vi "Final Project.vi"() -> ()   [LabVIEW 2022 SP3]
uses:
  <vilib>/Analysis/3filter.llb/Filter Passband Type.ctl
  <vilib>/Instr/_visa.llb/VISA Configure Serial Port (Instr).vi
  <vilib>/ptbypt/NI_PtbyPt.lvlib
  <vilib>/Analysis/NI_AALBase.lvlib
panel:
  out "EMG2":dbl
  out "EMG1":dbl
  in  "stop 3":bool
  out "Raw Data File":refnum<file>
  in  "stop 2":bool
  out "Folder_Name":string
  out "Jump Indicator":bool
  out "Jump Binary":dbl(graph)
  out "Left Indicator":bool
  out "Move Left Binary":dbl(graph)
  out "Voltage (Analog) 2":dbl(graph)
  out "Right Indicator":bool
  out "Move Right Binary":dbl(graph)
  out "Voltage (Analog)":dbl(graph)
  out "number":u32
  out "Index":i32
  out "read buffer":string
  out "Serial Settings:Number of Bytes at Serial Port":u32
  in  "stop":bool
  out "Available?":bool
  out "string":string
  in  "Knob":dbl(knob) scale=0.0..2.0
  in  "VISA resource name":refnum<visa-resource-name>
  in  "Baud Rate":u32=9600
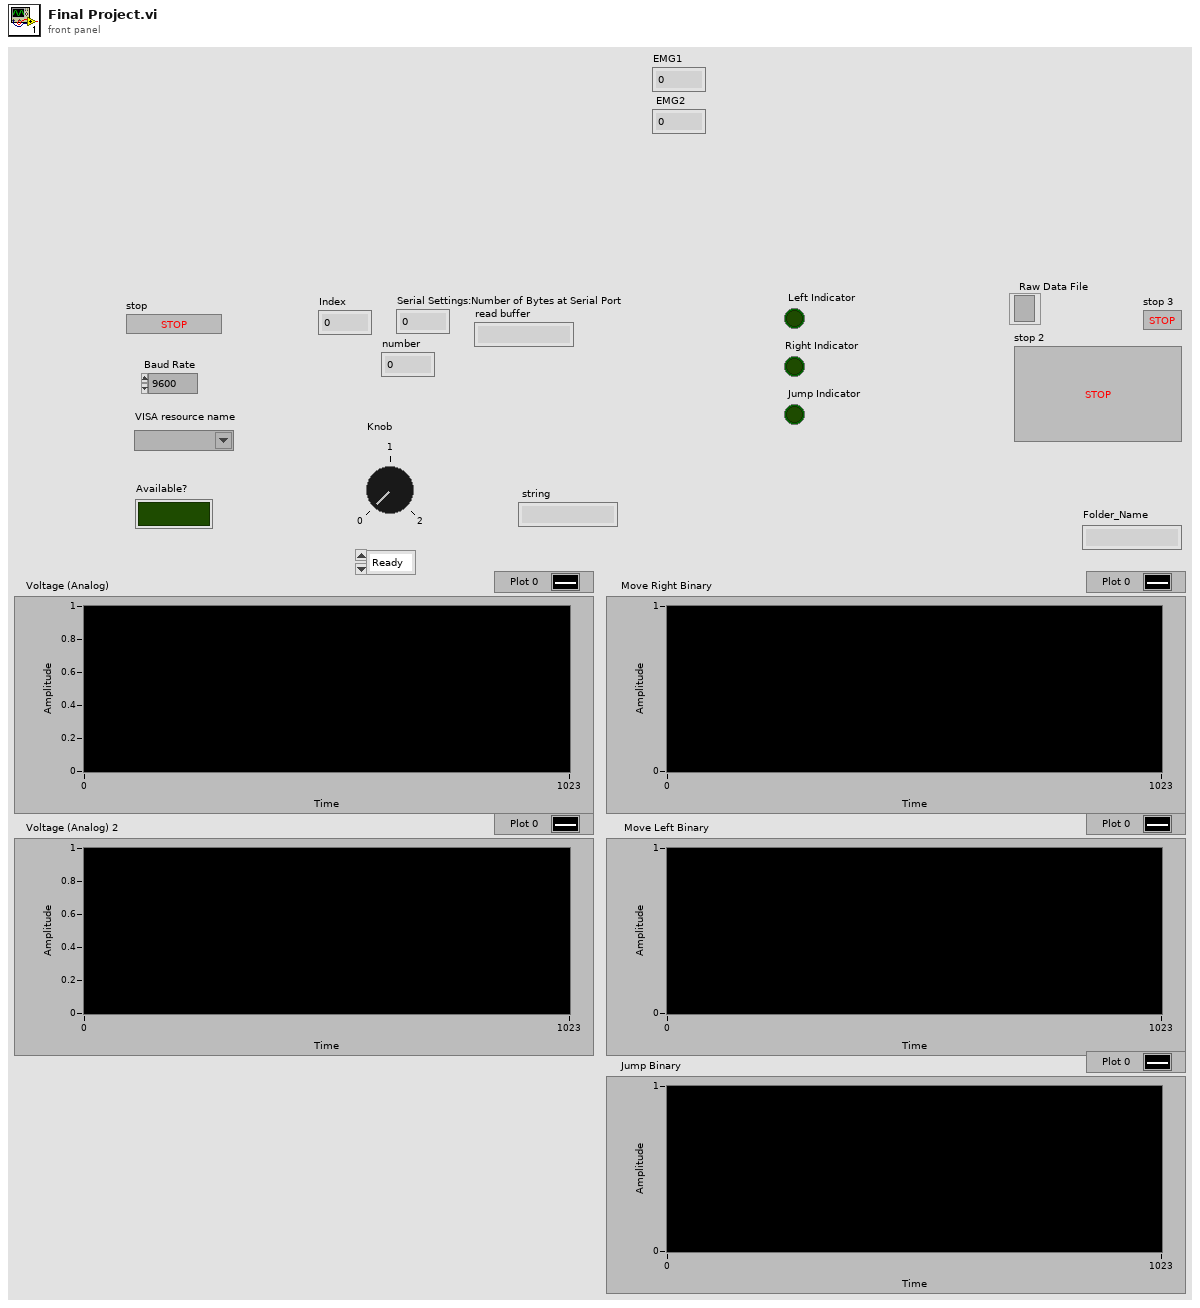
[diagram p1: front panel]
types:
  T1 = typedef "NI_AALBase.lvlib/Filter Passband Type.ctl" = enum32{"Lowpass", "Highpass", "Bandpass", "Bandstop"}
  T2 = enum16{"open", "replace", "create", "open or create", "replace or create", "replace or create with confirmation"}
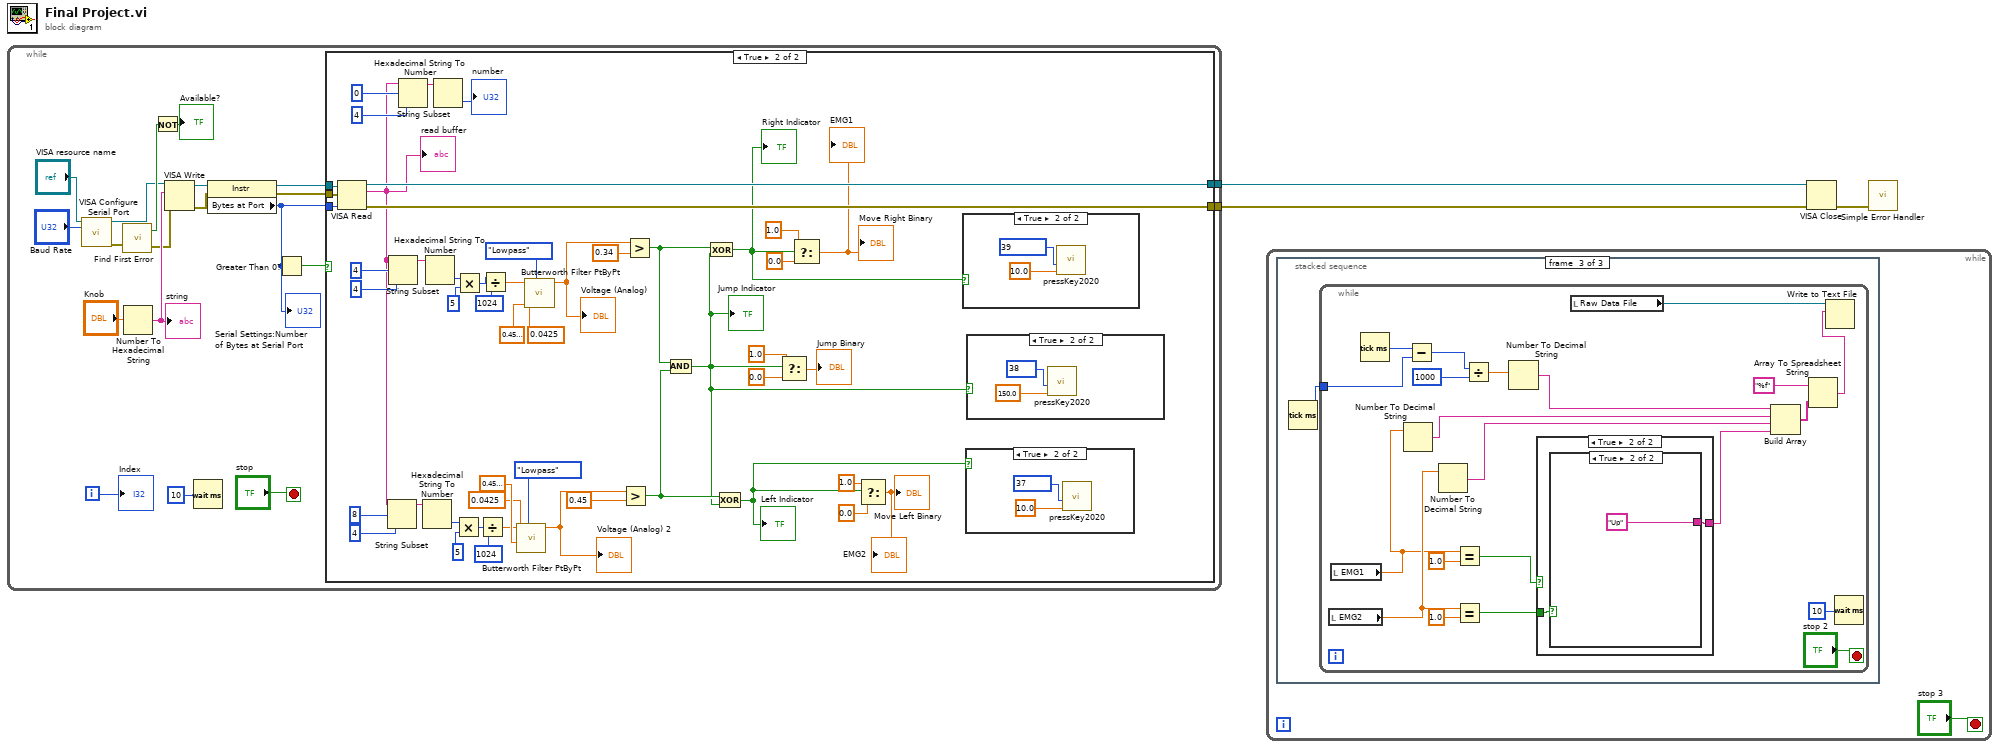
[diagram p0: block diagram]
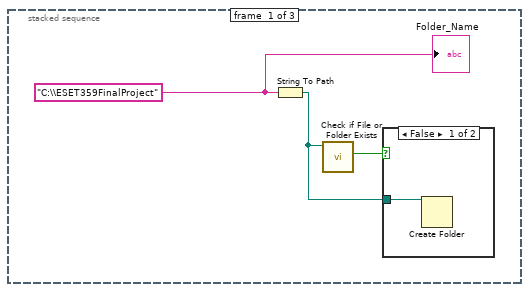
[diagram p2: hidden frame]
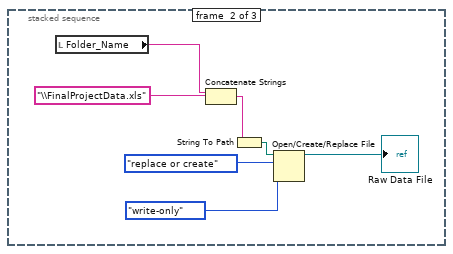
[diagram p4: hidden frame]
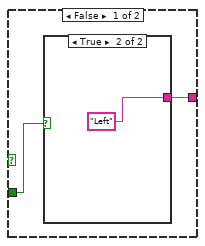
[diagram p5: hidden frame]
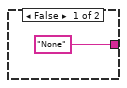
[diagram p6: hidden frame]
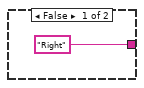
[diagram p7: hidden frame]
diagram:
  n1 = while {
    tunnel: [w6] -> w2
    tunnel: [w5] -> w1
    i -> [w4]
    stop <- "stop" stop-if-true
    n2 = call-poly "VISA Configure Serial Port"("VISA resource name"="VISA resource name", "baud rate (9600)"="Baud Rate") -> ("VISA resource name out"=w15:refnum<visa-resource-name>, "error out"=w21:errorcluster)  [unwired: 12 in]
    n3 = call <vilib>:"Find First Error.vi"("error in (no error)"=w21) -> ("error out"=w14:errorcluster, "error?"=w20:bool)  [unwired: 3 in]
    n4 = Number To Hexadecimal String(2:"Knob") -> (0:w16:string)  [unwired: 1 in]
    "string" <- w16
    n5 = Not(x=w20) -> (.not. x?=→"Available?":bool)
    n6 = VISA Write(VISA resource name=w15, write buffer=w16, error in (no error)=w14) -> (VISA resource name out=w13:refnum<visa-resource-name>, error out=w12:errorcluster)  [unwired: 1 out]
    n7 = Wait (ms)(milliseconds to wait=u32 10) -> ()  [unwired: 1 out]
    n8 = property class="Instr"(reference=w13, error in=w12) -> (reference out=w10:refnum<visa-resource-name>, error out=w11:errorcluster, "Bytes at Port"=w9:u32)
    "Serial Settings:Number of Bytes at Serial Port" <- w9
    n9 = Greater Than 0?(x=w9) -> (x > 0?=w8:bool)
    n10 = case shown="True" w8 {
      tunnel: w11 -> [w24 w75]
      tunnel: w9 -> [_ w74]
      tunnel: w10 -> [w25 w73]
      tunnel: [w25 w72] -> w5
      tunnel: [w24 w71] -> w6
      frame False {
      }
      frame True {
        n11 = VISA Read(VISA resource name=w73, byte count=w74, error in (no error)=w75) -> (VISA resource name out=w72:refnum<visa-resource-name>, read buffer=w41:string, error out=w71:errorcluster)  [unwired: 1 out]
        "read buffer" <- w41
        n12 = String Subset(string=w41, offset (0)=8, length (rest)=4 ("length (rest)")) -> (substring=w50:string)
        n13 = String Subset(string=w41, offset (0)=4, length (rest)=4 ("length (rest)")) -> (substring=w64:string)
        n14 = String Subset(string=w41, offset (0)=0, length (rest)=4 ("length (rest)")) -> (substring=w68:string)
        n15 = Hexadecimal String To Number(string=w50) -> (number=w49:u32)  [unwired: 2 in, 1 out]
        n16 = Hexadecimal String To Number(string=w64) -> (number=w63:u32)  [unwired: 2 in, 1 out]
        n17 = Hexadecimal String To Number(string=w68) -> (number=→"number":u32)  [unwired: 2 in, 1 out]
        n18 = Multiply(x=w49, y=u32 5) -> (x*y=w47:u32)
        n19 = Multiply(x=w63, y=u32 5) -> (x*y=w61:u32)
        n20 = Divide(x=w47, y=u32 1024) -> (x/y=w43:dbl)
        n21 = Divide(x=w61, y=u32 1024) -> (x/y=w54:dbl)
        n22 = call <vilib>:"Butterworth Filter PtByPt.vi"("filter type"=Filter_Passband_Type."Lowpass", "low cutoff freq: fl"=0.0425, "high cutoff freq: fh"=0.45000000000000007, "x"=w43) -> ("Filtered x"=w38:dbl)  [unwired: 5 in, 1 out]
        "Voltage (Analog) 2" <- w38
        n23 = call <vilib>:"Butterworth Filter PtByPt.vi"("filter type"=Filter_Passband_Type."Lowpass", "low cutoff freq: fl"=0.0425, "high cutoff freq: fh"=0.45000000000000007, "x"=w54) -> ("Filtered x"=w53:dbl)  [unwired: 5 in, 1 out]
        "Voltage (Analog)" <- w53
        n24 = Greater?(x=w38, y=0.45) -> (0:w29:bool)
        n25 = Greater?(x=w53, y=0.34) -> (0:w31:bool)
        n26 = And(x=w31, y=w29) -> (x .and. y?=w27:bool)
        "Jump Indicator" <- w27
        n27 = Exclusive Or(1:w27, 2:w31) -> (0:w30:bool)
        "Right Indicator" <- w30
        n28 = Exclusive Or(1:w27, 2:w29) -> (0:w28:bool)
        "Left Indicator" <- w28
        n29 = Select(t=1.0, s=w27, f=0.0) -> (s? t:f=→"Jump Binary":dbl)
        n30 = Select(t=1.0, s=w30, f=0.0) -> (s? t:f=→"Move Right Binary" →"EMG1":dbl)
        n31 = Select(t=1.0, s=w28, f=0.0) -> (s? t:f=→"Move Left Binary" →"EMG2":dbl)
        n32 = case shown="True" w30 {
          frame False {
          }
          frame True {
            n33 = call "pressKey2020.vi"("time"=10.0, "Virtual Key"=u8 39) -> ()  [unwired: 10 in]
          }
        }
        n34 = case shown="True" w28 {
          frame False {
          }
          frame True {
            n35 = call "pressKey2020.vi"("time"=10.0, "Virtual Key"=u8 37) -> ()  [unwired: 10 in]
          }
        }
        n36 = case shown="True" w27 {
          frame False {
          }
          frame True {
            n37 = call "pressKey2020.vi"("time"=150.0, "Virtual Key"=u8 38) -> ()  [unwired: 10 in]
          }
        }
      }
    }
    "Index" <- w4
  }
  n38 = while {
    stop <- "stop 3" stop-if-true
    n39 = stacked-sequence {
      frame #0 {
        w83 = "C:\\ESET359FinalProject"
        n40 = String To Path(string=w83) -> (path=w85:path)
        n41 = call <vilib>:"Check if File or Folder Exists.vi"("path"=w85) -> ("file or folder exists?"=w84:bool)  [unwired: 8 in, 2 out]
        n42 = case shown="False" w84 {
          tunnel: w85 -> [w86 _]
          frame False {
            n43 = Create Folder(path (use dialog)=w86) -> ()  [unwired: 2 in, 3 out]
          }
          frame True {
          }
        }
        "Folder_Name" <- w83
      }
      frame #1 {
        n44 = local read "Folder_Name"() -> (w88:string)
        n45 = Concatenate Strings(w88, "\\FinalProjectData.xls") -> (w92:string)
        n46 = String To Path(string=w92) -> (path=w91:path)
        n47 = Open/Create/Replace File(file path (use dialog)=w91, operation (0:open)=T2."replace or create" ("operation (0: Open)"), access (0:read/write)=enum16{"read/write", "read-only", "write-only"}."write-only") -> (refnum out=→"Raw Data File":refnum<file>)  [unwired: 3 in, 2 out]
      }
      frame #2 {
        n48 = Tick Count (ms)() -> (millisecond timer value=w94:u32)
        n49 = while {
          tunnel: w94 -> [w109]
          stop <- "stop 2" stop-if-true
          n50 = local read "EMG2"() -> (w97:dbl)
          n51 = local read "EMG1"() -> (w96:dbl)
          n52 = Tick Count (ms)() -> (millisecond timer value=w113:u32)
          n53 = Number To Decimal String(number=w96) -> (decimal integer string=w100:string)  [unwired: 1 in]
          n54 = Subtract(x=w113, y=w109) -> (x-y=w112:u32)
          n55 = Number To Decimal String(number=w97) -> (decimal integer string=w99:string)  [unwired: 1 in]
          n56 = Equal?(x=w96, y=1.0) -> (x = y?=w105:bool)
          n57 = Equal?(x=w97, y=1.0) -> (x = y?=w104:bool)
          n58 = Divide(x=w112, y=1000) -> (x/y=w102:dbl)
          n59 = Number To Decimal String(number=w102) -> (decimal integer string=w101:string)  [unwired: 1 in]
          n60 = case shown="True" w105 {
            tunnel: w104 -> [w117 w121]
            tunnel: [w116 w120] -> w103
            frame False {
              n61 = case shown="True" w117 {
                tunnel: ["None" "Left"] -> w116
                frame False {
                }
                frame True {
                }
              }
            }
            frame True {
              n62 = case shown="True" w121 {
                tunnel: ["Right" "Up"] -> w120
                frame False {
                }
                frame True {
                }
              }
            }
          }
          n63 = local read "Raw Data File"() -> (w98:refnum<file>)
          n64 = Build Array(w101, w100, w99, w103) -> (w110:string[])
          n65 = Array To Spreadsheet String(array=w110, 3:"%f") -> (spreadsheet string=w114:string)  [unwired: 1 in]
          n66 = Write to Text File(file (use dialog)=w98, text=w114) -> ()  [unwired: 2 in, 3 out]
          n67 = Wait (ms)(milliseconds to wait=u32 10) -> ()  [unwired: 1 out]
        }
      }
    }
  }
  n68 = VISA Close(VISA resource name=w1, error in (no error)=w2) -> (error out=w3:errorcluster)
  n69 = call <vilib>:"Simple Error Handler.vi"("error in (no error)"=w3) -> ()  [unwired: 4 in, 5 out]
